vi "MagnitudeCalc.vi"(3 "Y":dbl, 5 "X":dbl) -> (2 "sqrt(X^2+Y^2)":dbl)   [LabVIEW 2011]
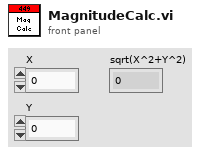
[diagram p1: front panel]
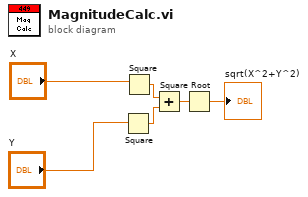
[diagram p0: block diagram]
diagram:
  n1 = Square(x="Y") -> (x^2=w2:dbl)
  n2 = Square(x="X") -> (x^2=w1:dbl)
  n3 = Add(x=w1, y=w2) -> (x+y=w3:dbl)
  n4 = Square Root(x=w3) -> (sqrt(x)=→"sqrt(X^2+Y^2)":dbl)
